vi "SPARC4_GUI.vi"() -> ()   [LabVIEW 2018]
uses:
  SPARC4_GUI/SPARC4_GUI.lvclass
  Stream/Stream.lvclass/Stream.ctl
  Interface/Interface.lvclass/Interface.ctl
  State Machine/State Machine.lvclass
  Stream/Stream.lvclass
  Interface/Interface.lvclass
panel:
  out "Error":string
  in  "Tab Control 2":enum32{"Front Panel", "Setup Panel"}(tab)
  out "CCD Status":string
  out "Current image":string="CH1"
  out "% Acquired":u16
  out "Exposing":bool
  out "Temperature 2":i16
  out "Serial Number":u16
  out "Temperature Status":string
  in  "Base Name":string="CH1"
  in  "Exp Time 2":sgl=1e-05 min=1e-05
  in  "# Images":u32=1 min=1
  out "Exposições realizadas":u8(slide) max=2 scale=0.0..1.0
  in  "Acquire":bool
  in  "Command:":string
  out "Response:":string
  out "Initialization":bool
  in  "SEND":bool
  in  "IP Address:":string="//localhost"
  in  "Night Directory:":string="C:\\Users\\observer\\Desktop\\Imagens\\"
  in  "Stop Application":bool
  in  "Shutter Mode":u8(ring)=2 items=["Fully Auto", "OPEN", "CLOSED"]
  in  "Kinetic Series Length":u16=1 min=1
  in  "Cooler ON/OFF":u16(ring) items=["Cooler OFF", "Cooler ON"]
  in  "Temperature":i16=20 min=-80 max=20
  in  "Exposure Time":sgl=1e-05 min=1e-05
  in  "Readout Rate":u8(ring) items=["30 MHz", "20 MHz", "10 MHz", "  1 MHz"]
  in  "Pre-amp gain":u8(ring) items=["Gain 1", "Gain 2"]
  in  "EM Gain":u16=2
  in  "EM Mode":u8(ring) items=["Electron Multiplying", "Conventional"]
  in  "Sub Image":T1(radio)=enum."1024 x 1024"
  in  "Final Line":u16=1024
  in  "Final Column":u16=1024
  in  "Initial Cloumn":u16=1
  in  "Initial Line":u16=1
  in  "Binning":u16=1
  # "SPARC4 \nGeneral User Interface (GUI)"
  # "Command Acquisition Control"
  # "Channel 1: acquisition control & status"
  # "Temperature & Shutter"
  # "Timings"
  # "Horizontal pixel shift"
  # "EM Mode"
  # "Sub Image & Binning"
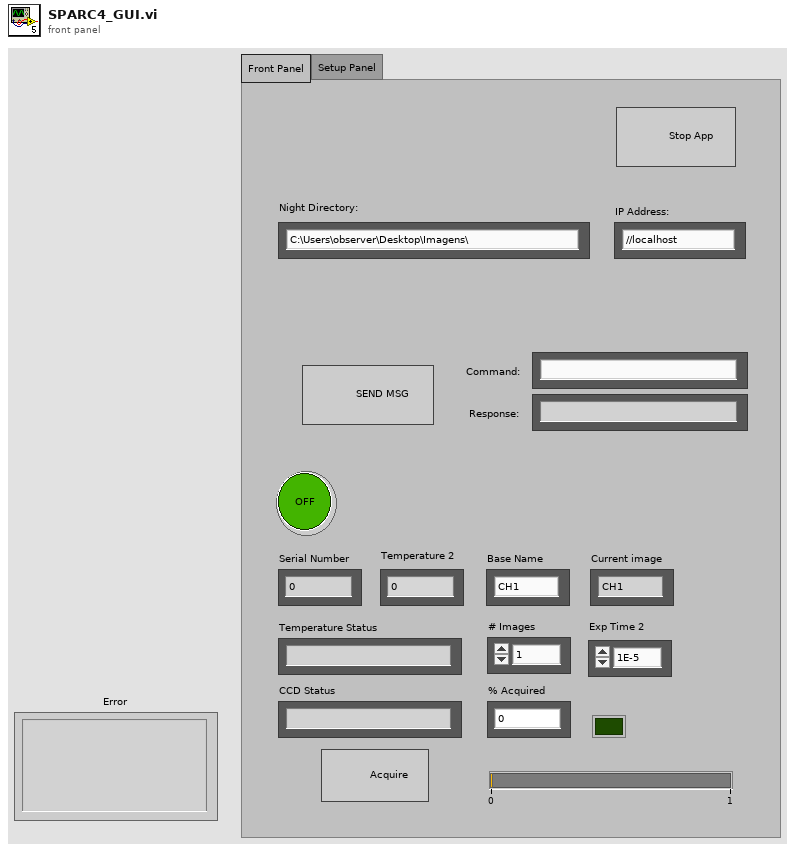
[diagram p1: front panel]
types:
  T1 = enum32{"256 x 256", "512 x 512", "1024 x 1024", "Custom"}
  T2 = cluster{"Exposure Time":sgl, "Pre-amp gain":u8, "Readout Rate":u8, "EM Mode":u8, "EM Gain":u16, "Binning":u16, "Initial Line":u16, "Initial Cloumn":u16, "Final Line":u16, "Final Column":u16, "Kinetic Series Length":u32, "Shutter Mode":u8, "Cooler ON/OFF":u16, "Temperature":i8, "Image Name":string, "Image Path":string, "# Images":u32}
  T3 = cluster{"% Acquired":u16, "Acquiring":bool, "Current image name":string, "Current sequence":u16, "CCD State":string}
  T4 = cluster{"Initialization":bool, "Serial Number":u16}
  T5 = cluster{"Current Temperature":i16, "Temperatue Status":string}
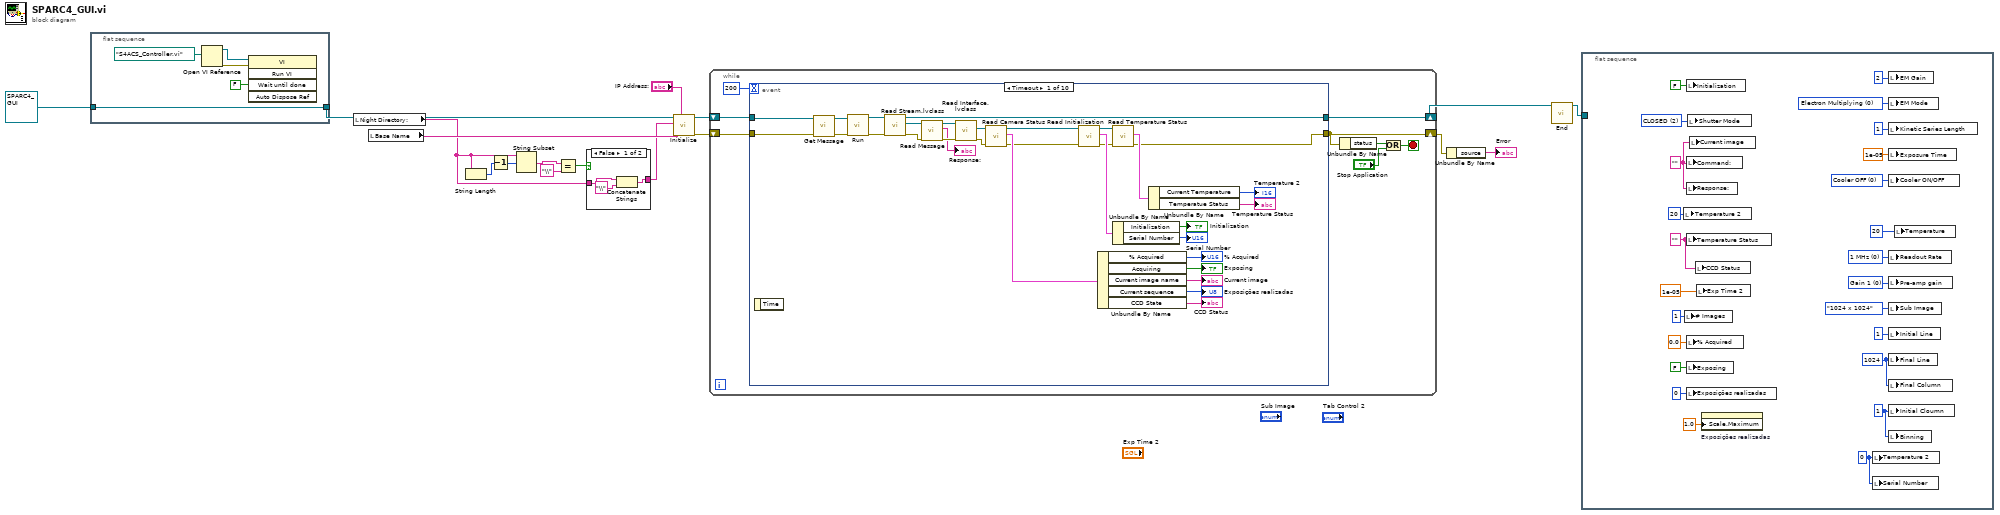
[diagram p0: block diagram]
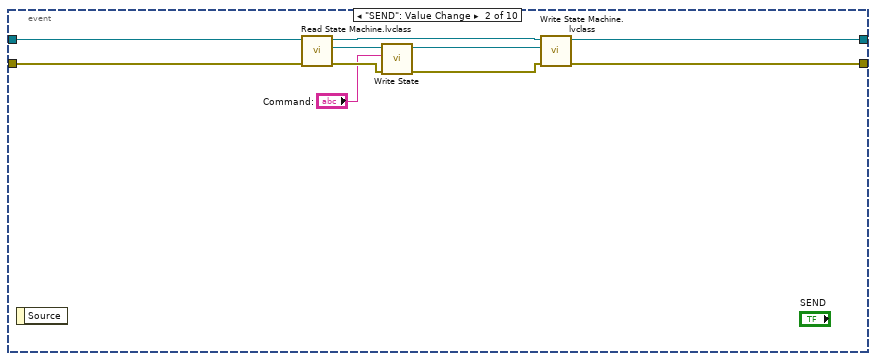
[diagram p3: hidden frame]
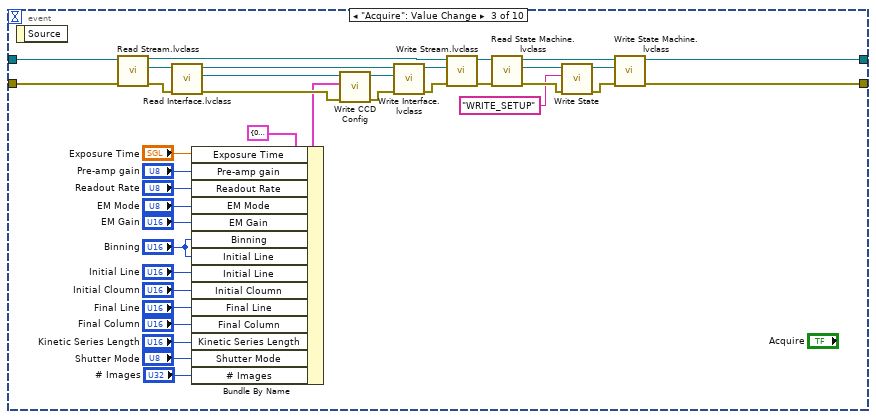
[diagram p4: hidden frame]
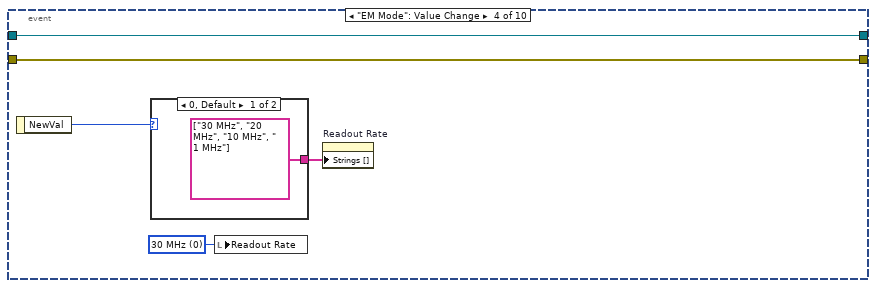
[diagram p5: hidden frame]
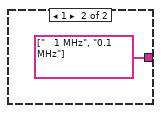
[diagram p6: hidden frame]
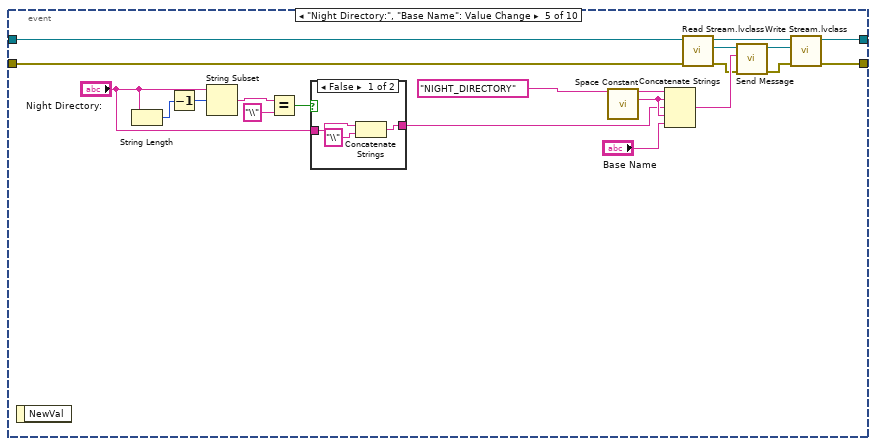
[diagram p7: hidden frame]
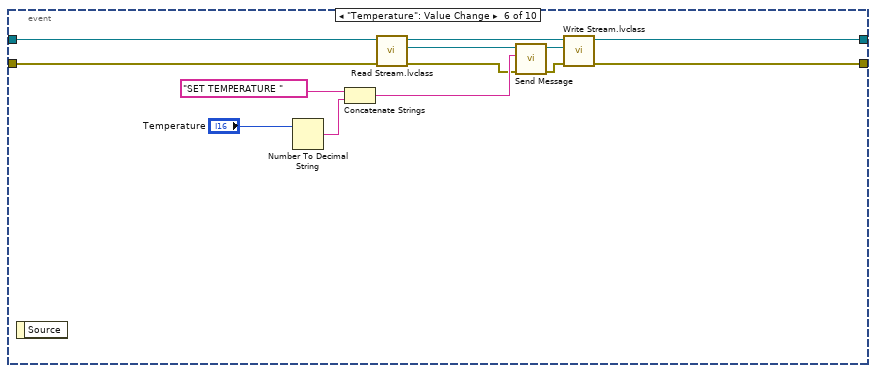
[diagram p9: hidden frame]
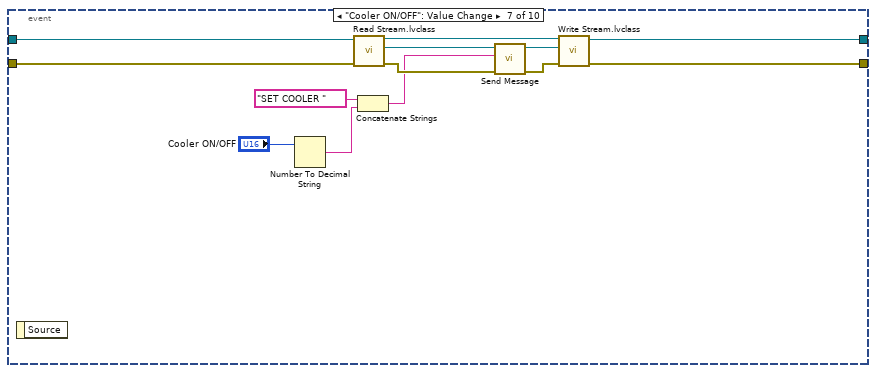
[diagram p10: hidden frame]
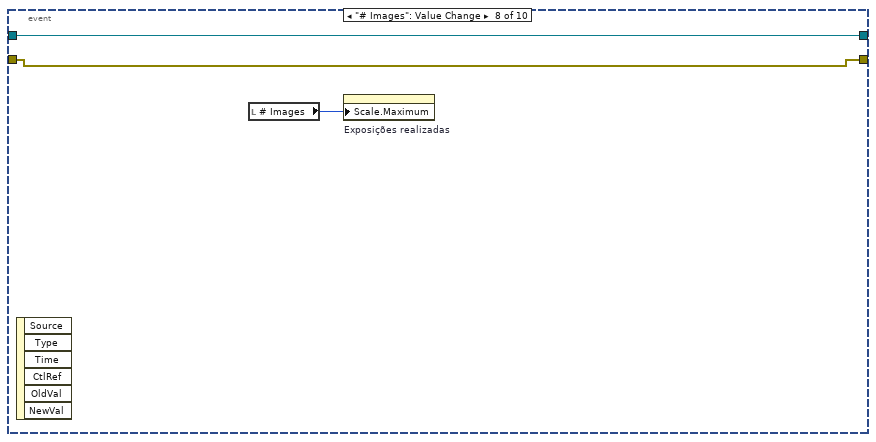
[diagram p11: hidden frame]
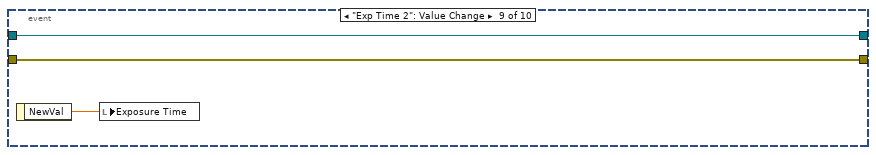
[diagram p12: hidden frame]
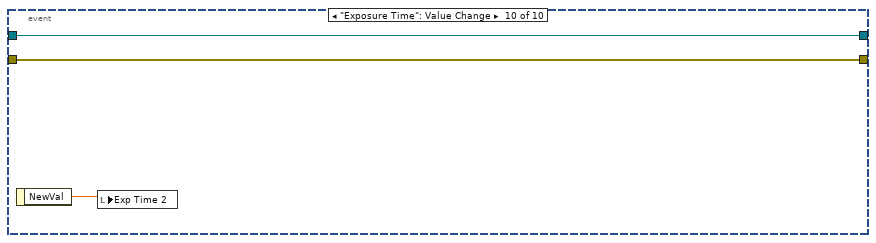
[diagram p13: hidden frame]
diagram:
  n1 = flat-sequence {
    tunnel: refnum<class "SPARC4_GUI.lvclass"> refnum ("SPARC4_GUI.lvclass") -> [w18]
    tunnel: [w18] -> w15
    frame #0 {
      n2 = Open VI Reference(vi path=path "S4ACS_Controller.vi") -> (vi reference=w22:refnum<vi>, error out=w21:errorcluster)  [unwired: 5 in]
      n3 = invoke class="VI" method="Run VI"(reference=w22, error in=w21, "Wait until done"=FALSE ("Wait Until Done")) -> ()  [unwired: 2 in, 5 out]
    }
  }
  n4 = local read "Night Directory:"() -> (w2:string)
  n5 = local read "Base Name"() -> (w12:string)
  n6 = String Length(string=w2) -> (length=w6:i32)
  n7 = Decrement(x=w6) -> (x-1=w5:i32)
  n8 = String Subset(string=w2, offset (0)=w5) -> (substring=w4:string)  [unwired: 1 in]
  n9 = Equal?(x=w4, y="\\") -> (x = y?=w3:bool)
  n10 = case shown="False" w3 {
    tunnel: [w25 w26] -> w1
    tunnel: w2 -> [w23 w26]
    frame False {
      n11 = Concatenate Strings(w23, "\\") -> (w25:string)
    }
    frame True {
    }
  }
  n12 = call "Initialize.vi"("IP"="IP Address:", "Image Name"=w12, "Night Directory:"=w1, "SPARC4_GUI in"=w15) -> ("error out"=w17:errorcluster, "SPARC4_GUI out"=w16:refnum<class "SPARC4_GUI.lvclass">)  [unwired: 6 in]
  n13 = while {
    shift-right: [w27] -> w9
    shift-left: w17 -> [w28]
    shift-right: [w30] -> w10
    shift-left: w16 -> [w29]
    stop <- w33 stop-if-true
    n14 = event shown="[0] Timeout" {
      selector: _ -> [_ _ _ _ _ _ _ _ _ _]
      dyn-events: _ -> [_ _ _ _ _ _ _ _ _ _]
      timeout: 200 -> [_ _ _ _ _ _ _ _ _ _]
      tunnel: w28 -> [w55 w74 w96 w116 w127 w148 w162 w171 w174 w177]
      tunnel: [w43 w66 w86 w116 w132 w145 w168 w171 w174 w177] -> w27
      tunnel: w29 -> [w56 w75 w97 w117 w128 w149 w161 w172 w175 w176]
      tunnel: [w54 w67 w87 w117 w133 w144 w169 w172 w175 w176] -> w30
      event Timeout {
        n15 = event-data() -> ()  [unwired: 1 in, 1 out]
        n16 = call "Get Message.vi"("error in (no error)"=w55, "SPARC4_GUI in"=w56) -> ("error out"=w58:errorcluster, "SPARC4_GUI out"=w57:refnum<class "SPARC4_GUI.lvclass">)  [unwired: 8 in]
        n17 = call "Run.vi"("error in (no error)"=w58, "SPARC4_GUI in"=w57) -> ("error out"=w63:errorcluster, "SPARC4_GUI out"=w62:refnum<class "SPARC4_GUI.lvclass">)  [unwired: 8 in]
        n18 = call "Read Stream.lvclass.vi"("error in (no error)"=w63, "SPARC4_GUI in"=w62) -> ("error out"=w39:errorcluster, "Stream.lvclass"=w42:refnum<class "Stream.lvclass">, "SPARC4_GUI out"=w54:refnum<class "SPARC4_GUI.lvclass">)  [unwired: 7 in]
        n19 = call "Read Message.vi"("error in (no error)"=w39, "Stream in"=w42) -> ("error out"=w40:errorcluster, "Message"=→"Response:":string, "Stream out"=w41:refnum<class "Stream.lvclass">)  [unwired: 7 in]
        n20 = call "Read Interface.lvclass.vi"("error in (no error)"=w40, "Stream in"=w41) -> ("error out"=w60:errorcluster, "Interface.lvclass"=w61:refnum<class "Interface.lvclass">)  [unwired: 7 in, 1 out]
        n21 = call "Read Camera Status.vi"("error in (no error)"=w60, "Interface in"=w61) -> ("error out"=w53:errorcluster, "Camera Status"=w59:T3, "Interface out"=w52:refnum<class "Interface.lvclass">)  [unwired: 7 in]
        n22 = call "Read Initialization.vi"("error in (no error)"=w53, "Interface in"=w52) -> ("error out"=w48:errorcluster, "Initialization"=w51:T4, "Interface out"=w47:refnum<class "Interface.lvclass">)  [unwired: 7 in]
        n23 = Unbundle By Name(w59) -> ("% Acquired"=→"% Acquired":u16, "Acquiring"=→"Exposing":bool, "Current image name"=→"Current image":string, "Current sequence"=→"Exposições realizadas":u16, "CCD State"=→"CCD Status":string)
        n24 = call "Read Temperature Status.vi"("error in (no error)"=w48, "Interface in"=w47) -> ("error out"=w43:errorcluster, "Temperature Status"=w46:T5)  [unwired: 7 in, 1 out]
        n25 = Unbundle By Name(w51) -> ("Initialization"=→"Initialization":bool, "Serial Number"=→"Serial Number":u16)
        n26 = Unbundle By Name(w46) -> ("Current Temperature"=→"Temperature 2":i16, "Temperatue Status"=→"Temperature Status":string)
      }
      event "SEND": Value Change {
        n27 = event-data() -> ()  [unwired: 1 in, 1 out]
        n28 = call "Read State Machine.lvclass.vi"("error in (no error)"=w74, "SPARC4_GUI in"=w75) -> ("error out"=w70:errorcluster, "State Machine.lvclass"=w73:refnum<class "State Machine.lvclass">, "SPARC4_GUI out"=w69:refnum<class "SPARC4_GUI.lvclass">)  [unwired: 7 in]
        n29 = call-dynamic "Write State.vi"("error in (no error)"=w70, "State"="Command:", "State Machine in"=w73) -> ("error out"=w71:errorcluster, "State Machine out"=w72:refnum<class "State Machine.lvclass">)  [unwired: 7 in]
        n30 = call "Write State Machine.lvclass.vi"("error in (no error)"=w71, "State Machine.lvclass"=w72, "SPARC4_GUI in"=w69) -> ("error out"=w66:errorcluster, "SPARC4_GUI out"=w67:refnum<class "SPARC4_GUI.lvclass">)  [unwired: 7 in]
      }
      event "Acquire": Value Change {
        n31 = event-data() -> ()  [unwired: 1 in, 1 out]
        n32 = call "Read Stream.lvclass.vi"("error in (no error)"=w96, "SPARC4_GUI in"=w97) -> ("error out"=w93:errorcluster, "Stream.lvclass"=w94:refnum<class "Stream.lvclass">, "SPARC4_GUI out"=w95:refnum<class "SPARC4_GUI.lvclass">)  [unwired: 7 in]
        n33 = call "Read Interface.lvclass.vi"("error in (no error)"=w93, "Stream in"=w94) -> ("error out"=w111:errorcluster, "Interface.lvclass"=w112:refnum<class "Interface.lvclass">, "Stream out"=w98:refnum<class "Stream.lvclass">)  [unwired: 7 in]
        n34 = Bundle By Name(cluster=T2 {"Exposure Time"=0.0, "Pre-amp gain"=0, "Readout Rate"=0, "EM Mode"=0, "EM Gain"=2, "Binning"=1, "Initial Line"=1, "Initial Cloumn"=1, "Final Line"=1024, "Final Column"=1024, "Kinetic Series Length"=0, "Shutter Mode"=2, "Cooler ON/OFF"=0, "Temperature"=20, "Image Name"="", "Image Path"="", "# Images"=1} ("CCD Config"), "Exposure Time"="Exposure Time", "Pre-amp gain"="Pre-amp gain", "Readout Rate"="Readout Rate", "EM Mode"="EM Mode", "EM Gain"="EM Gain", "Binning"="Binning", "Initial Line"="Binning", "Initial Line"="Initial Line", "Initial Cloumn"="Initial Cloumn", "Final Line"="Final Line", "Final Column"="Final Column", "Kinetic Series Length"="Kinetic Series Length", "Shutter Mode"="Shutter Mode", "# Images"="# Images") -> (w110:T2)
        n35 = call "Write CCD Config.vi"("error in (no error)"=w111, "CCD Config"=w110, "Interface in"=w112) -> ("error out"=w77:errorcluster, "Interface out"=w76:refnum<class "Interface.lvclass">)  [unwired: 7 in]
        n36 = call "Write Interface.lvclass.vi"("error in (no error)"=w77, "Interface.lvclass"=w76, "Stream in"=w98) -> ("error out"=w91:errorcluster, "Stream out"=w92:refnum<class "Stream.lvclass">)  [unwired: 7 in]
        n37 = call "Write Stream.lvclass.vi"("error in (no error)"=w91, "Stream.lvclass"=w92, "SPARC4_GUI in"=w95) -> ("error out"=w90:errorcluster, "SPARC4_GUI out"=w89:refnum<class "SPARC4_GUI.lvclass">)  [unwired: 7 in]
        n38 = call "Read State Machine.lvclass.vi"("error in (no error)"=w90, "SPARC4_GUI in"=w89) -> ("error out"=w82:errorcluster, "State Machine.lvclass"=w85:refnum<class "State Machine.lvclass">, "SPARC4_GUI out"=w88:refnum<class "SPARC4_GUI.lvclass">)  [unwired: 7 in]
        n39 = call-dynamic "Write State.vi"("error in (no error)"=w82, "State"="WRITE_SETUP", "State Machine in"=w85) -> ("error out"=w83:errorcluster, "State Machine out"=w84:refnum<class "State Machine.lvclass">)  [unwired: 7 in]
        n40 = call "Write State Machine.lvclass.vi"("error in (no error)"=w83, "State Machine.lvclass"=w84, "SPARC4_GUI in"=w88) -> ("error out"=w86:errorcluster, "SPARC4_GUI out"=w87:refnum<class "SPARC4_GUI.lvclass">)  [unwired: 7 in]
      }
      event "EM Mode": Value Change {
        w113 = u8 0 items=["30 MHz", "20 MHz", "10 MHz", "1 MHz"] ("Readout Rate")
        n41 = event-data() -> ("NewVal"=w114:u8)  [unwired: 1 in]
        n42 = case shown="0, Default" w114 {
          tunnel: [string[] ["30 MHz", "20 MHz", "10 MHz", "  1 MHz"] string[] ["   1 MHz", "0.1 MHz"]] -> w115
          frame 0, Default {
          }
          frame 1 {
          }
        }
        n43 = local write "Readout Rate"(w113) -> ()
        n44 = property on="Readout Rate" class="Ring (strict)"("Strings []"=w115) -> ()  [unwired: 2 in, 2 out]
      }
      event "Night Directory:", "Base Name": Value Change {
        n45 = event-data() -> ()  [unwired: 1 in, 1 out]
        n46 = String Length(string="Night Directory:") -> (length=w122:i32)
        n47 = Decrement(x=w122) -> (x-1=w123:i32)
        n48 = String Subset(string="Night Directory:", offset (0)=w123) -> (substring=w124:string)  [unwired: 1 in]
        n49 = Equal?(x=w124, y="\\") -> (x = y?=w125:bool)
        n50 = case shown="False" w125 {
          tunnel: [w142 w143] -> w120
          tunnel: "Night Directory:" -> [w140 w143]
          frame False {
            n51 = Concatenate Strings(w140, "\\") -> (w142:string)
          }
          frame True {
          }
        }
        n52 = call <vilib>:"Space Constant.vi"() -> ("String"=w137:string)
        n53 = Concatenate Strings("NIGHT_DIRECTORY" ("Message"), w137, w120, w137, "Base Name") -> (w138:string)
        n54 = call "Read Stream.lvclass.vi"("error in (no error)"=w127, "SPARC4_GUI in"=w128) -> ("error out"=w130:errorcluster, "Stream.lvclass"=w131:refnum<class "Stream.lvclass">, "SPARC4_GUI out"=w129:refnum<class "SPARC4_GUI.lvclass">)  [unwired: 7 in]
        n55 = call "Send Message.vi"("error in (no error)"=w130, "Message"=w138, "Stream in"=w131) -> ("error out"=w135:errorcluster, "Stream out"=w134:refnum<class "Stream.lvclass">)  [unwired: 7 in]
        n56 = call "Write Stream.lvclass.vi"("error in (no error)"=w135, "Stream.lvclass"=w134, "SPARC4_GUI in"=w129) -> ("error out"=w132:errorcluster, "SPARC4_GUI out"=w133:refnum<class "SPARC4_GUI.lvclass">)  [unwired: 7 in]
      }
      event "Temperature": Value Change {
        n57 = event-data() -> ()  [unwired: 1 in, 1 out]
        n58 = Number To Decimal String(number="Temperature") -> (decimal integer string=w154:string)  [unwired: 1 in]
        n59 = Concatenate Strings("SET TEMPERATURE " ("Message"), w154) -> (w155:string)
        n60 = call "Read Stream.lvclass.vi"("error in (no error)"=w148, "SPARC4_GUI in"=w149) -> ("error out"=w147:errorcluster, "Stream.lvclass"=w152:refnum<class "Stream.lvclass">, "SPARC4_GUI out"=w150:refnum<class "SPARC4_GUI.lvclass">)  [unwired: 7 in]
        n61 = call "Send Message.vi"("error in (no error)"=w147, "Message"=w155, "Stream in"=w152) -> ("error out"=w146:errorcluster, "Stream out"=w151:refnum<class "Stream.lvclass">)  [unwired: 7 in]
        n62 = call "Write Stream.lvclass.vi"("error in (no error)"=w146, "Stream.lvclass"=w151, "SPARC4_GUI in"=w150) -> ("error out"=w145:errorcluster, "SPARC4_GUI out"=w144:refnum<class "SPARC4_GUI.lvclass">)  [unwired: 7 in]
      }
      event "Cooler ON/OFF": Value Change {
        n63 = event-data() -> ()  [unwired: 1 in, 1 out]
        n64 = Number To Decimal String(number="Cooler ON/OFF") -> (decimal integer string=w158:string)  [unwired: 1 in]
        n65 = call "Read Stream.lvclass.vi"("error in (no error)"=w162, "SPARC4_GUI in"=w161) -> ("error out"=w164:errorcluster, "Stream.lvclass"=w163:refnum<class "Stream.lvclass">, "SPARC4_GUI out"=w167:refnum<class "SPARC4_GUI.lvclass">)  [unwired: 7 in]
        n66 = Concatenate Strings("SET COOLER ", w158) -> (w157:string)
        n67 = call "Send Message.vi"("error in (no error)"=w164, "Message"=w157, "Stream in"=w163) -> ("error out"=w165:errorcluster, "Stream out"=w166:refnum<class "Stream.lvclass">)  [unwired: 7 in]
        n68 = call "Write Stream.lvclass.vi"("error in (no error)"=w165, "Stream.lvclass"=w166, "SPARC4_GUI in"=w167) -> ("error out"=w168:errorcluster, "SPARC4_GUI out"=w169:refnum<class "SPARC4_GUI.lvclass">)  [unwired: 7 in]
      }
      event "# Images": Value Change {
        n69 = event-data() -> ()  [unwired: 1 in, 6 out]
        n70 = local read "# Images"() -> (w170:u32)
        n71 = property on="Exposições realizadas" class="Slide (strict)"("Scale.Maximum"=w170) -> ()  [unwired: 2 in, 2 out]
      }
      event "Exp Time 2": Value Change {
        n72 = event-data() -> ("NewVal"=w173:sgl)  [unwired: 1 in]
        n73 = local write "Exposure Time"(w173) -> ()
      }
      event "Exposure Time": Value Change {
        n74 = event-data() -> ("NewVal"=w178:sgl)  [unwired: 1 in]
        n75 = local write "Exp Time 2"(w178) -> ()
      }
    }
    n76 = Unbundle By Name(w27) -> ("status"=w32:bool)
    n77 = Or(x=w32, y="Stop Application") -> (x .or. y?=w33:bool)
  }
  n78 = Unbundle By Name(w9) -> ("source"=→"Error":string)
  n79 = call "End.vi"("SPARC4_GUI in"=w10) -> ("SPARC4_GUI out"=w11:refnum<class "SPARC4_GUI.lvclass">)  [unwired: 9 in, 1 out]
  n80 = flat-sequence {
    tunnel: w11 -> [_]
    frame #0 {
      w179 = i16 0 ("Temperature 2")
      w183 = u8 2 items=["Fully Auto", "OPEN", "CLOSED"] ("Shutter Mode")
      w180 = "" ("Command:")
      w185 = u16 1024 ("Final Line")
      w184 = u16 1 ("Initial Cloumn")
      w188 = u8 0 items=["Gain 1", "Gain 2"] ("Pre-amp gain")
      w189 = u8 0 items=["1 MHz", "10 MHz", "20 MHz", "30 MHz"] ("Readout Rate")
      w191 = u16 0 items=["Cooler OFF", "Cooler ON"] ("Cooler ON/OFF")
      w194 = u8 0 items=["Electron Multiplying", "Conventional"] ("EM Mode")
      w181 = "" ("Temperature Status")
      n81 = local write "Temperature 2"(20 ("Temperature")) -> ()
      n82 = local write "# Images"(u32 1 ("# Ciclos")) -> ()
      n83 = local write "Initialization"(FALSE ("Initialization")) -> ()
      n84 = local write "Command:"(w180) -> ()
      n85 = local write "Response:"(w180) -> ()
      n86 = local write "Temperature Status"(w181) -> ()
      n87 = local write "% Acquired"(0.0 ("% Acquired")) -> ()
      n88 = local write "Exposing"(FALSE ("Exposing")) -> ()
      n89 = local write "Exposições realizadas"(u8 0 ("Exposições realizadas")) -> ()
      n90 = local write "Shutter Mode"(w183) -> ()
      n91 = local write "Current image"(w180) -> ()
      n92 = local write "CCD Status"(w181) -> ()
      n93 = local write "Exp Time 2"(1e-05 ("Exposure Time 2")) -> ()
      n94 = property on="Exposições realizadas" class="Slide (strict)"("Scale.Maximum"=1.0 ("Scale.Range:Maximum")) -> ()  [unwired: 2 in, 2 out]
      n95 = local write "Temperature 2"(w179) -> ()
      n96 = local write "Serial Number"(w179) -> ()
      n97 = local write "EM Gain"(u16 2 ("EM Gain")) -> ()
      n98 = local write "EM Mode"(w194) -> ()
      n99 = local write "Kinetic Series Length"(u16 1 ("Kinetic Series Length")) -> ()
      n100 = local write "Exposure Time"(1e-05 ("Exposure Time")) -> ()
      n101 = local write "Cooler ON/OFF"(w191) -> ()
      n102 = local write "Readout Rate"(w189) -> ()
      n103 = local write "Pre-amp gain"(w188) -> ()
      n104 = local write "Sub Image"(T1."1024 x 1024" ("Sub Image")) -> ()
      n105 = local write "Initial Line"(u16 1 ("Initial Line")) -> ()
      n106 = local write "Final Line"(w185) -> ()
      n107 = local write "Final Column"(w185) -> ()
      n108 = local write "Initial Cloumn"(w184) -> ()
      n109 = local write "Binning"(w184) -> ()
      n110 = local write "Temperature"(i16 20 ("Set temperature")) -> ()
    }
  }
